vi "Dynamic Channel Lookups.vi"(8 "error in (no error)":errorcluster, 11 "Child Refs":T1[](array[typedef]) format="%.0x") -> (0 "error out":errorcluster, 3 "SLSC Dynamic Inputs":T2[](array[typedef]))   [LabVIEW 2015, in "SLSC Module Template System Explorer.lvlib"]
uses:
  SLSC Module Template System Explorer.lvlib
  Shared/SLSC Dynamic Channel.ctl
  <vilib>/NI Veristand/Custom Device API/Custom Device Item Ref.ctl
  Shared/Constants.vi
  <vilib>/NI Veristand/Custom Device API/Get Item Property (String).vi
  <vilib>/regexp/Match Regular Expression.xnode
  <vilib>/NI Veristand/Custom Device API/Custom Device API.lvlib
  Shared/SLSC Module Template Shared.lvlib
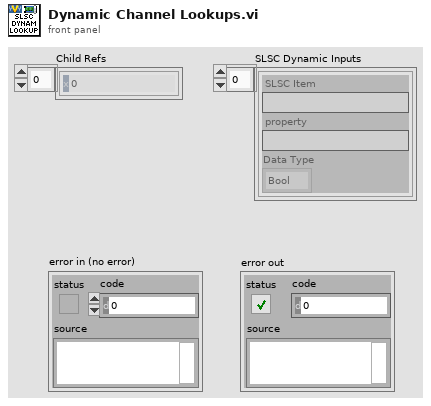
[diagram p1: front panel]
types:
  T1 = typedef "Custom Device API.lvlib/Custom Device Item Ref.ctl" = u64
  T2 = typedef "SLSC Module Template System Explorer.lvlib/SLSC Dynamic Channel.ctl" = cluster{"SLSC Item":string, "property":string, "Data Type":enum16{"Bool", "Double", "I32", "I64", "String", "U32", "U64"}}
  T3 = enum16{"Bool", "Double", "I32", "I64", "String", "U32", "U64"}
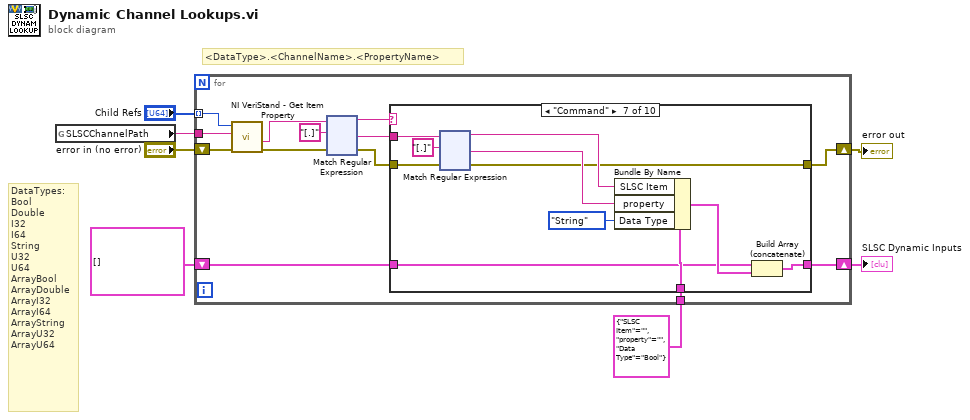
[diagram p0: block diagram]
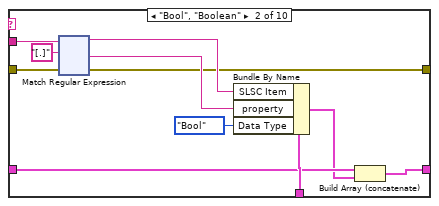
[diagram p3: hidden frame]
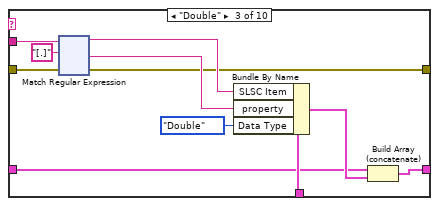
[diagram p4: hidden frame]
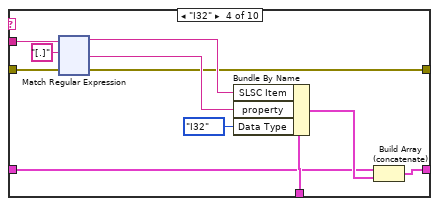
[diagram p5: hidden frame]
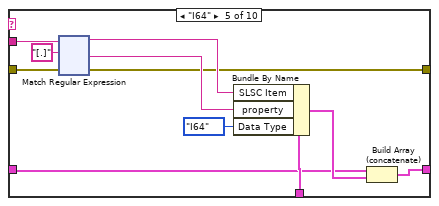
[diagram p6: hidden frame]
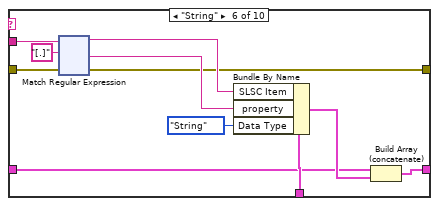
[diagram p7: hidden frame]
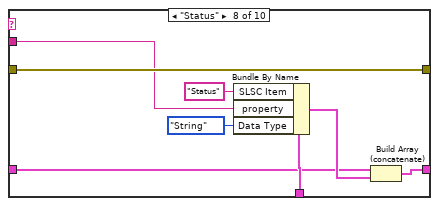
[diagram p8: hidden frame]
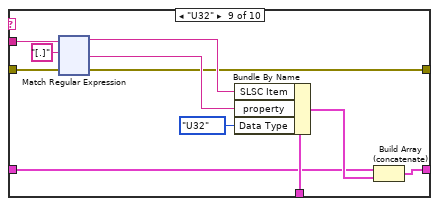
[diagram p9: hidden frame]
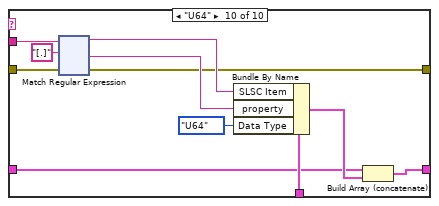
[diagram p10: hidden frame]
diagram:
  # "<DataType>.<ChannelName>.<PropertyName>"
  # "DataTypes:\nBool\nDouble\nI32\nI64\nString\nU32\nU64\nArrayBool\nArrayDouble\nArrayI32\nArrayI64\nArrayString\nArrayU32\nArrayU64"
  n1 = global read "Constants.vi" "SLSCChannelPath"() -> (w6:string)
  n2 = for {
    tunnel: "Child Refs" -> [w20] mode=indexing
    tunnel: w6 -> [w19]
    shift-right: [w8] -> w1
    shift-left: "error in (no error)" -> [w14]
    tunnel: T2 {"SLSC Item"="", "property"="", "Data Type"=enum."Bool"} ("SLSC Dynamic Channel") -> [w11]
    shift-right: [w9] -> w2
    shift-left: T2[] [] ("SLSC Dynamic Inputs") -> [w10]
    n3 = call-poly <vilib>:"NI VeriStand - Get Item Property.vi"("error in (no error)"=w14, "Property Name"=w19, "Item Ref in"=w20) -> ("error out"=w12:errorcluster, "Value"=w13:string)  [unwired: 5 in, 2 out]
    n4 = xnode "Match Regular Expression"("input string"=w13, "regular expression"="[.]", "error in"=w12) -> ("before match"=w16:string, "after match"=w17:string, "error out"=w18:errorcluster)  [unwired: 3 in, 2 out]
    n5 = case shown="\"Command\"" w16 {
      tunnel: w17 -> [_ w32 w157 w282 w407 w532 w657 w774 w790 w915]
      tunnel: w18 -> [w22 w31 w156 w281 w406 w531 w656 w775 w789 w914]
      tunnel: w11 -> [_ w28 w151 w278 w403 w528 w653 w780 w786 w911]
      tunnel: w10 -> [w21 w27 w149 w275 w399 w525 w650 w777 w782 w907]
      tunnel: [w21 w26 w152 w274 w400 w524 w649 w776 w784 w908] -> w9
      tunnel: [w22 w24 w148 w273 w398 w523 w648 w775 w781 w906] -> w8
      frame Default {
      }
      frame "Bool", "Boolean" {
        n6 = xnode "Match Regular Expression"("input string"=w32, "regular expression"="[.]", "error in"=w31) -> ("before match"=w30:string, "after match"=w29:string, "error out"=w24:errorcluster)  [unwired: 3 in, 2 out]
        n7 = Bundle By Name(cluster=w28, "SLSC Item"=w30, "property"=w29, "Data Type"=T3."Bool") -> (w25:T2)
        n8 = Build Array (concatenate)(w27, w25) -> (w26:T2[])
      }
      frame "Double" {
        n9 = xnode "Match Regular Expression"("input string"=w157, "regular expression"="[.]", "error in"=w156) -> ("before match"=w155:string, "after match"=w154:string, "error out"=w148:errorcluster)  [unwired: 3 in, 2 out]
        n10 = Bundle By Name(cluster=w151, "SLSC Item"=w155, "property"=w154, "Data Type"=T3."Double") -> (w150:T2)
        n11 = Build Array (concatenate)(w149, w150) -> (w152:T2[])
      }
      frame "I32" {
        n12 = xnode "Match Regular Expression"("input string"=w282, "regular expression"="[.]", "error in"=w281) -> ("before match"=w280:string, "after match"=w279:string, "error out"=w273:errorcluster)  [unwired: 3 in, 2 out]
        n13 = Bundle By Name(cluster=w278, "SLSC Item"=w280, "property"=w279, "Data Type"=T3."I32") -> (w276:T2)
        n14 = Build Array (concatenate)(w275, w276) -> (w274:T2[])
      }
      frame "I64" {
        n15 = xnode "Match Regular Expression"("input string"=w407, "regular expression"="[.]", "error in"=w406) -> ("before match"=w405:string, "after match"=w404:string, "error out"=w398:errorcluster)  [unwired: 3 in, 2 out]
        n16 = Bundle By Name(cluster=w403, "SLSC Item"=w405, "property"=w404, "Data Type"=T3."I64") -> (w401:T2)
        n17 = Build Array (concatenate)(w399, w401) -> (w400:T2[])
      }
      frame "String" {
        n18 = xnode "Match Regular Expression"("input string"=w532, "regular expression"="[.]", "error in"=w531) -> ("before match"=w530:string, "after match"=w529:string, "error out"=w523:errorcluster)  [unwired: 3 in, 2 out]
        n19 = Bundle By Name(cluster=w528, "SLSC Item"=w530, "property"=w529, "Data Type"=T3."String") -> (w526:T2)
        n20 = Build Array (concatenate)(w525, w526) -> (w524:T2[])
      }
      frame "Command" {
        n21 = xnode "Match Regular Expression"("input string"=w657, "regular expression"="[.]", "error in"=w656) -> ("before match"=w655:string, "after match"=w654:string, "error out"=w648:errorcluster)  [unwired: 3 in, 2 out]
        n22 = Bundle By Name(cluster=w653, "SLSC Item"=w655, "property"=w654, "Data Type"=T3."String") -> (w651:T2)
        n23 = Build Array (concatenate)(w650, w651) -> (w649:T2[])
      }
      frame "Status" {
        n24 = Bundle By Name(cluster=w780, "SLSC Item"="Status", "property"=w774, "Data Type"=T3."String") -> (w778:T2)
        n25 = Build Array (concatenate)(w777, w778) -> (w776:T2[])
      }
      frame "U32" {
        n26 = xnode "Match Regular Expression"("input string"=w790, "regular expression"="[.]", "error in"=w789) -> ("before match"=w788:string, "after match"=w787:string, "error out"=w781:errorcluster)  [unwired: 3 in, 2 out]
        n27 = Bundle By Name(cluster=w786, "SLSC Item"=w788, "property"=w787, "Data Type"=T3."U32") -> (w783:T2)
        n28 = Build Array (concatenate)(w782, w783) -> (w784:T2[])
      }
      frame "U64" {
        n29 = xnode "Match Regular Expression"("input string"=w915, "regular expression"="[.]", "error in"=w914) -> ("before match"=w913:string, "after match"=w912:string, "error out"=w906:errorcluster)  [unwired: 3 in, 2 out]
        n30 = Bundle By Name(cluster=w911, "SLSC Item"=w913, "property"=w912, "Data Type"=T3."U64") -> (w909:T2)
        n31 = Build Array (concatenate)(w907, w909) -> (w908:T2[])
      }
    }
  }
  "SLSC Dynamic Inputs" <- w2
  "error out" <- w1
